vi "AD5933_Config2RegisterData (SubVI).vi"(0 "AD5933 Configuration":T2={"Start Frequency / Hz"=0.0, "Frequency Increment / Hz"=0.1, "Number of Increments / #"=0, "Number of Setting Time Cycles / # "=0, "Exitation Voltage"=enum."2V", "PGA Gain"=enum."5x"} {"Number of Setting Time Cycles / #" max=2044 step=1; "Number of Increments / #" max=511; "Frequency Increment / Hz" min=0.1 max=100000.0 step=0.1 format="%#_6p"; "Start Frequency / Hz" min=0.0 max=100000.0 step=0.1 format="%#_6p"}) -> (1 "FrequencySweepConfigArray (Reg 0x82-0x8B)":T1, 2 "ConfigRegister (0x80)":u8)   [LabVIEW 2017]
uses:
  TypeDefs/AD5933_Config.ctl
  TypeDefs/AD5933_FreqSweepConfigRegisterArray.ctl
panel:
  out "0x80":u8 format="%08b"
  out "0x8A":u8 format="%02x"
  out "0x8B":u8 format="%02x"
  out "0x89":u8 format="%02x"
  out "0x88":u8 format="%02x"
  out "0x85":u8 format="%02x"
  out "0x86":u8 format="%02x"
  out "0x87":u8 format="%02x"
  out "0x84":u8 format="%02x"
  out "0x83":u8 format="%02x"
  out "0x82":u8 format="%02x"
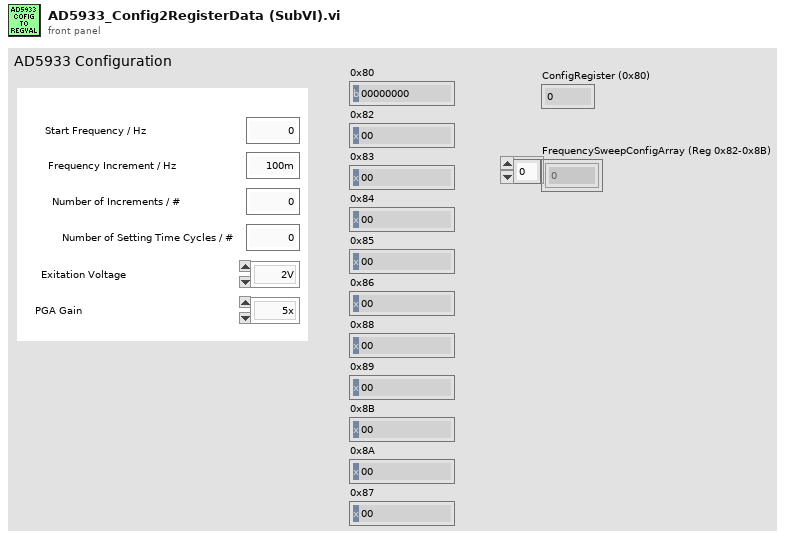
[diagram p1: front panel]
types:
  T1 = typedef "AD5933_FreqSweepConfigRegisterArray.ctl" = u8[]
  T2 = typedef "AD5933_Config.ctl" = cluster{"Start Frequency / Hz":dbl, "Frequency Increment / Hz":dbl, "Number of Increments / #":u16, "Number of Setting Time Cycles / # ":u16, "Exitation Voltage":enum8{"2V", "200mV", "400mV", "1V"}, "PGA Gain":enum8{"5x", "1x"}}
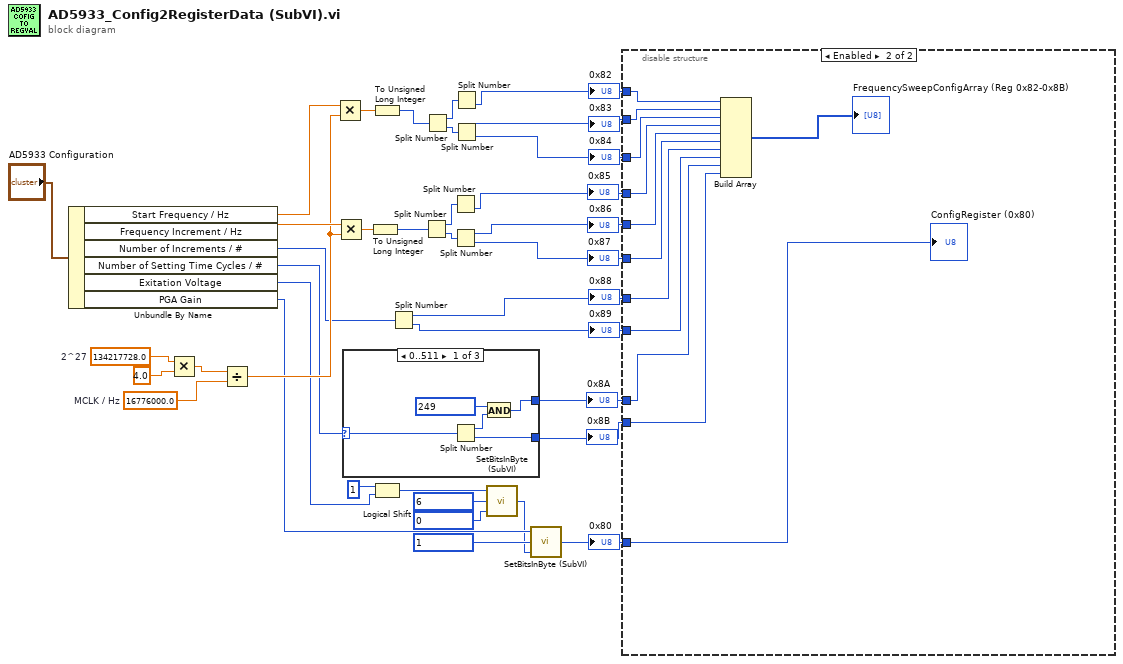
[diagram p0: block diagram]
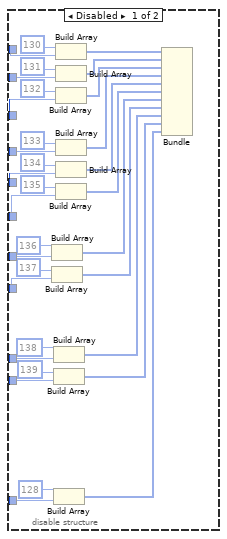
[diagram p2: hidden frame]
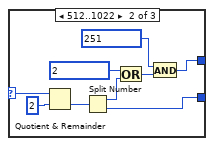
[diagram p3: hidden frame]
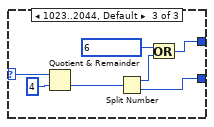
[diagram p4: hidden frame]
diagram:
  w33 = 16776000.0  # MCLK / Hz
  w36 = 134217728.0  # 2^27
  n1 = Unbundle By Name("AD5933 Configuration") -> ("Start Frequency / Hz"=w32:dbl, "Frequency Increment / Hz"=w31:dbl, "Number of Increments / #"=w21:u16, "Number of Setting Time Cycles / #"=w20:u16, "Exitation Voltage"=w12:enum8{"2V", "200mV", "400mV", "1V"}, "PGA Gain"=w16:enum8{"5x", "1x"})
  n2 = Multiply(x=w36, y=4.0 ("2^27")) -> (x*y=w34:dbl)
  n3 = Divide(x=w34, y=w33) -> (x/y=w30:dbl)
  n4 = Multiply(x=w32, y=w30) -> (x*y=w29:dbl)
  n5 = Multiply(x=w31, y=w30) -> (x*y=w25:dbl)
  n6 = case shown="0..511" w20 {
    selector: w20 -> [w42 w51 w54]
    tunnel: [w39 w44 w52] -> w3
    tunnel: [w38 w43 w53] -> w2
    frame 0..511 {
      n7 = Split Number(x=w42) -> (hi(x)=w40:u8, lo(x)=w38:u8)
      n8 = And(x=u8 249 ("0x85"), y=w40) -> (x .and. y?=w39:u8)
    }
    frame 512..1022 {
      n9 = Quotient & Remainder(x=w51, y=u16 2) -> (floor(x/y)=w49:u16)  [unwired: 1 out]
      n10 = Split Number(x=w49) -> (hi(x)=w48:u8, lo(x)=w43:u8)
      n11 = Or(x=u8 2 ("0x85"), y=w48) -> (x .or. y?=w45:u8)
      n12 = And(x=u8 251 ("0x85"), y=w45) -> (x .and. y?=w44:u8)
    }
    frame 1023..2044, Default {
      n13 = Quotient & Remainder(x=w54, y=u16 4) -> (floor(x/y)=w58:u16)  [unwired: 1 out]
      n14 = Split Number(x=w58) -> (hi(x)=w57:u8, lo(x)=w53:u8)
      n15 = Or(x=u8 6 ("0x85"), y=w57) -> (x .or. y?=w52:u8)
    }
  }
  "0x8B" <- w2
  "0x8A" <- w3
  n16 = To Unsigned Long Integer(number=w25) -> (unsigned 32bit integer=w22:u32)
  n17 = To Unsigned Long Integer(number=w29) -> (unsigned 32bit integer=w28:u32)
  n18 = Logical Shift(y=u8 1, x=w12) -> (x << y=w14:u32)
  n19 = Split Number(x=w21) -> (hi(x)=w5:u8, lo(x)=w4:u8)
  "0x88" <- w5
  "0x89" <- w4
  n20 = Split Number(x=w22) -> (hi(x)=w23:u16, lo(x)=w24:u16)
  n21 = Split Number(x=w28) -> (hi(x)=w27:u16, lo(x)=w26:u16)
  n22 = Split Number(x=w23) -> (lo(x)=w8:u8)  [unwired: 1 out]
  "0x85" <- w8
  n23 = Split Number(x=w24) -> (hi(x)=w7:u8, lo(x)=w6:u8)
  "0x86" <- w7
  "0x87" <- w6
  n24 = Split Number(x=w27) -> (lo(x)=w11:u8)  [unwired: 1 out]
  "0x82" <- w11
  n25 = Split Number(x=w26) -> (hi(x)=w10:u8, lo(x)=w9:u8)
  "0x83" <- w10
  "0x84" <- w9
  n26 = call "SetBitsInByte (SubVI).vi"("Iput Byte"=u8 0 ("0x85"), "Bitsmask"=u8 6 ("0x85"), "Bits to set"=w14) -> ("Output Byte"=w15:u8)
  n27 = call "SetBitsInByte (SubVI).vi"("Iput Byte"=w15, "Bitsmask"=u8 1 ("0x85"), "Bits to set"=w16) -> ("Output Byte"=w1:u8)
  "0x80" <- w1
  n28 = disable-structure shown="Enabled" {
    disable-tunnel: w11 -> [w91 w103]
    disable-tunnel: w10 -> [w87 w102]
    disable-tunnel: w9 -> [w85 w101]
    disable-tunnel: w8 -> [w81 w100]
    disable-tunnel: w7 -> [w80 w99]
    disable-tunnel: w6 -> [w79 w98]
    disable-tunnel: w5 -> [w77 w97]
    disable-tunnel: w4 -> [w76 w96]
    disable-tunnel: w3 -> [w72 w95]
    disable-tunnel: w2 -> [w71 w94]
    disable-tunnel: w1 -> [w69 w92]
    frame Disabled {
      n29 = Build Array(u8 136 ("element"), w77) -> (w62:u8[])
      n30 = Build Array(u8 137 ("element"), w76) -> (w61:u8[])
      n31 = Build Array(u8 138 ("element"), w72) -> (w60:u8[])
      n32 = Build Array(u8 139 ("element"), w71) -> (w59:u8[])
      n33 = Build Array(u8 128 ("element"), w69) -> (w66:u8[])
      n34 = Build Array(u8 130 ("element"), w91) -> (w89:u8[])
      n35 = Build Array(u8 131 ("element"), w87) -> (w68:u8[])
      n36 = Build Array(u8 132 ("element"), w85) -> (w67:u8[])
      n37 = Build Array(u8 133 ("element"), w81) -> (w65:u8[])
      n38 = Build Array(u8 134 ("element"), w80) -> (w64:u8[])
      n39 = Build Array(u8 135 ("element"), w79) -> (w63:u8[])
      n40 = Bundle(w89, w68, w67, w65, w64, w63, w62, w61, w60, w59, w66) -> ()  [unwired: 1 in, 1 out]
    }
    frame Enabled {
      n41 = Build Array(w103, w102, w101, w100, w99, w98, w97, w96, w95, w94) -> (→"FrequencySweepConfigArray (Reg 0x82-0x8B)":u8[])
      "ConfigRegister (0x80)" <- w92
    }
  }
